vi "Command_Turret_AutoTarget.vi"(7 "Startup":bool, 8 "Timeout":dbl, 9 "Kd":dbl=0.001, 10 "Ki":dbl=1e-05, 11 "Kp":dbl=0.06) -> (2 "Turret_Speed":dbl, 4 "Reint":bool, 6 "Completed":bool)   [LabVIEW 2019]
uses:
  Auto Utilities/Command_Execution_State.ctl
  Globals/Sensor_Values.vi
panel:
  in  "Acceptable_Error":dbl
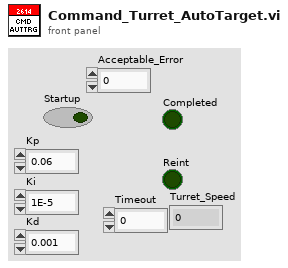
[diagram p1: front panel]
types:
  T1 = typedef "Command_Execution_State.ctl" = enum16{"Initialize", "Execute", "Finish"}
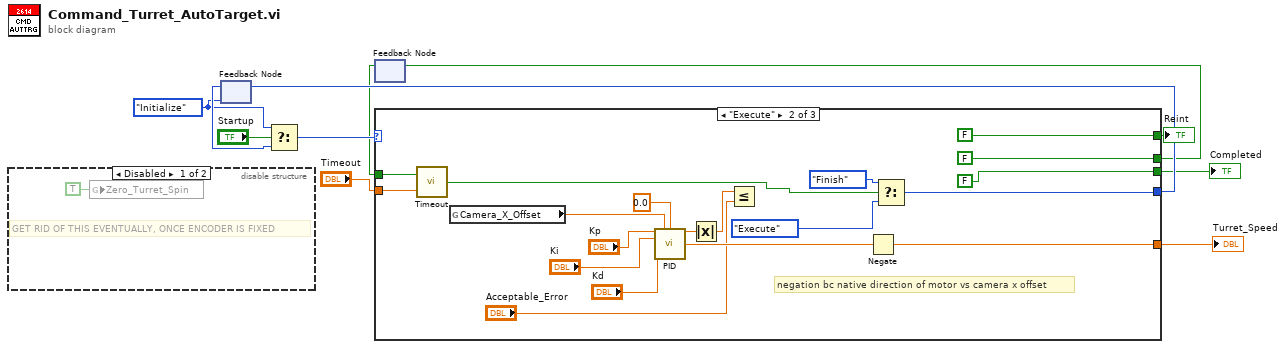
[diagram p0: block diagram]
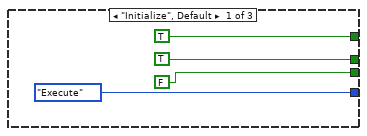
[diagram p3: hidden frame]
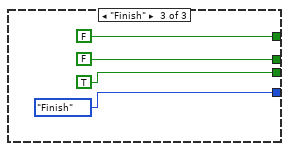
[diagram p4: hidden frame]
diagram:
  w5 = Command_Execution_State."Initialize" ("Play State")
  n1 = disable-structure shown="Disabled" {
    frame Disabled {
      # "GET RID OF THIS EVENTUALLY, ONCE ENCODER IS FIXED"
      n2 = global write "Sensor_Values.vi" "Zero_Turret_Spin"(TRUE ("Zero_Turret_Spin")) -> ()
    }
    frame Enabled {
    }
  }
  n3 = feedback #1(w5) -> (w9:T1)
  n4 = Select(t=w5, s="Startup", f=w9) -> (s? t:f=w11:T1)
  n5 = feedback #2() -> (w3:bool)  [unwired: 1 in]
  n6 = case shown="\"Execute\"" w11 {
    tunnel: [Command_Execution_State."Execute" ("Play State") w27 Command_Execution_State."Finish" ("Play State")] -> w10
    tunnel: [FALSE FALSE TRUE] -> w8
    tunnel: [TRUE FALSE FALSE] -> w6
    tunnel: w3 -> [_ w31 _]
    tunnel: [TRUE FALSE FALSE] -> w4
    tunnel: "Timeout" -> [_ w29 _]
    tunnel: [_ w18 _] -> w1
    frame "Initialize", Default {
    }
    frame "Execute" {
      # "negation bc native direction of motor vs camera x offset"
      n7 = call "Timeout.vi"("Timeout"=w29, "Initialize"=w31) -> ("Timed Out?"=w17:bool)
      n8 = global read "Sensor_Values.vi" "Camera_X_Offset"() -> (w33:dbl)
      n9 = call "PID.vi"("Kp"="Kp", "Process Variable"=w33, "Goal"=0.0, "Ki"="Ki", "Kd"="Kd") -> ("Current Error"=w24:dbl, "Command"=w25:dbl)  [unwired: 8 in, 1 out]
      n10 = Absolute Value(x=w24) -> (abs(x)=w23:dbl)
      n11 = Less Or Equal?(x=w23, y="Acceptable_Error") -> ()  [unwired: 1 out]
      n12 = Negate(x=w25) -> (-x=w18:dbl)
      n13 = Select(t=Command_Execution_State."Finish" ("Play State"), s=w17, f=Command_Execution_State."Execute" ("Play State")) -> (s? t:f=w27:T1)
    }
    frame "Finish" {
    }
  }
  "Completed" <- w8
  "Reint" <- w6
  "Turret_Speed" <- w1
  n14 = feedback-in #1(w10) -> ()
  n15 = feedback-in #2(w4) -> ()
